vi "Close.vi"(8 "error in (no error)":errorcluster, 11 "KST101 in":refnum<class "KST101.lvclass">) -> (0 "error out":errorcluster)   [LabVIEW 2016, in "Stepper Motor Controller.lvlib" / "KST101.lvclass"]
uses:
  KST101.lvclass
  KST101.lvclass/KST101.ctl
  D:/Workspace/ProCyteOne_LaserModuleAlignment/shared/Thorlabs/Kinesis/Dependencies/Thorlabs.MotionControl.KCube.StepperMotorCLI.dll
  Dependencies/Thorlabs.MotionControl.KCube.StepperMotorCLI.dll
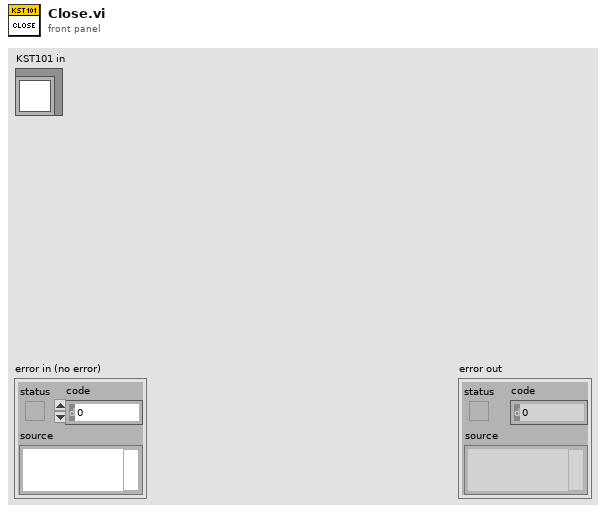
[diagram p1: front panel]
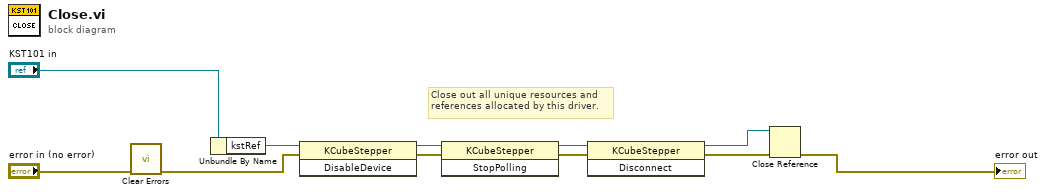
[diagram p0: block diagram]
diagram:
  # "Close out all unique resources and\nreferences allocated by this driver."
  n1 = call <vilib>:"Clear Errors.vi"("error in (no error)"="error in (no error)") -> ("error out"=w1:errorcluster)  [unwired: 5 in, 1 out]
  n2 = Unbundle By Name("KST101 in") -> ("kstRef"=w9:refnum<k24>)
  n3 = invoke class="KCubeStepper" method="DisableDevice"(reference=w9, error in=w1) -> (reference out=w6:refnum<k24>, error out=w4:errorcluster)  [unwired: 1 in, 1 out]
  n4 = invoke class="KCubeStepper" method="StopPolling"(reference=w6, error in=w4) -> (reference out=w5:refnum<k24>, error out=w3:errorcluster)  [unwired: 1 in, 1 out]
  n5 = invoke class="KCubeStepper" method="Disconnect"(reference=w5, error in=w3) -> (reference out=w8:refnum<k24>, error out=w7:errorcluster)  [unwired: 1 in, 1 out]
  n6 = Close Reference(reference=w8, error in (no error)=w7) -> (error out=→"error out":errorcluster)
